vi "VISP Snippet Write.vi"(8 "error in (no error)":errorcluster, 9 "Image Data in":T1, 10 "VI Path (*.vi)":path, 11 "VI Snippet Path (*.png)":path) -> (0 "error out":errorcluster)   [LabVIEW 2019, in "VI Snippet.lvlib"]
doc: "Writes the <b>VI Snippet Path (*.png)</b> image to disk including the embedded <b>VI Path (*.vi)</b> specified (as the \"niVI\" PNG chunk).\n\nCreated by: Ryan Pacini"
uses:
  VI Snippet.lvlib
  <vilib>/picture/picture.llb/imagedata.ctl
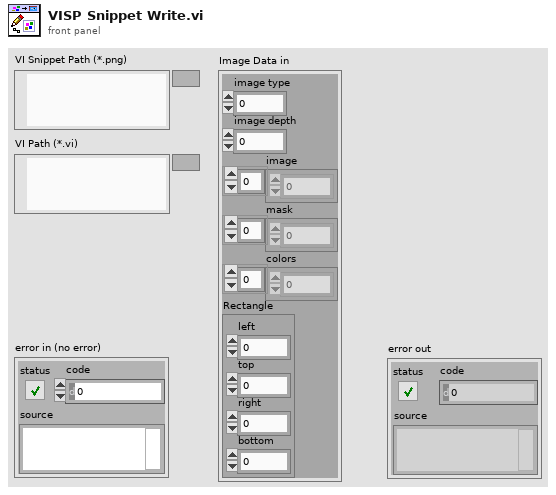
[diagram p1: front panel]
types:
  T1 = typedef "imagedata.ctl" = cluster{"image type":i32, "image depth":i32, "image":u8[], "mask":u8[], "colors":u32[], "Rectangle":cluster{"left":i16, "top":i16, "right":i16, "bottom":i16}}
  T2 = typedef "VI Snippet.lvlib/VISP PNG Chunk.ctl" = cluster{"Length":i32, "Type":string, "Data":string, "CRC":u32}
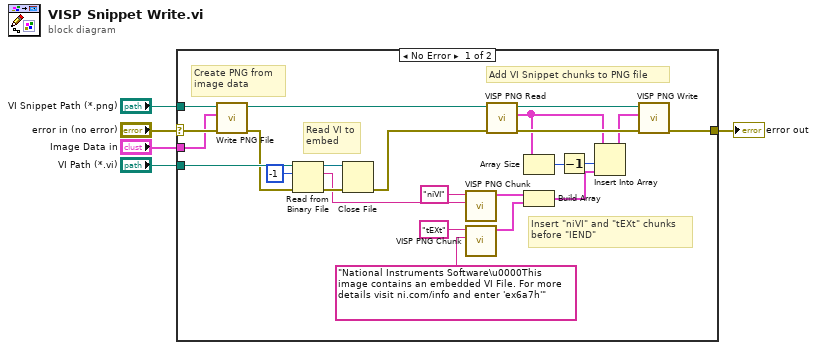
[diagram p0: block diagram]
diagram:
  n1 = case shown="No Error" "error in (no error)" {
    selector: "error in (no error)" -> [w29 w30]
    tunnel: "VI Snippet Path (*.png)" -> [w28 _]
    tunnel: "Image Data in" -> [w27 _]
    tunnel: [w16 w30] -> w3
    tunnel: "VI Path (*.vi)" -> [w15 _]
    frame No Error {
      # "Read VI to\nembed"
      # "Create PNG from\nimage data"
      # "Add VI Snippet chunks to PNG file"
      # "Insert \"niVI\" and \"tEXt\" chunks\nbefore \"IEND\""
      n2 = call <vilib>:"Write PNG File.vi"("error in (no error)"=w29, "image data"=w27, "path to PNG file"=w28) -> ("error out"=w11:errorcluster, "path"=w8:path)  [unwired: 7 in]
      n3 = Read from Binary File(8:w11, 10:-1 ("count (1)"), 11:w15) -> (0:w13:errorcluster, 2:w9:string, 3:w12:refnum<file>)  [unwired: 3 in, 1 out]
      n4 = Close File(refnum=w12, error in=w13) -> (error out=w10:errorcluster)  [unwired: 1 out]
      n5 = call "VISP PNG Chunk.vi"("Data"=w9, "Type"="niVI") -> ("PNG Chunk"=w19:T2)  [unwired: 9 in]
      n6 = call "VISP PNG Chunk.vi"("Data"="National Instruments Software\u0000This image contains an embedded VI File. For more details visit ni.com/info and enter 'ex6a7h'", "Type"="tEXt") -> ("PNG Chunk"=w18:T2)  [unwired: 9 in]
      n7 = call "VISP PNG Read.vi"("error in (no error)"=w10, "Image Path (*.png)"=w8) -> ("error out"=w26:errorcluster, "Chunks"=w7:T2[], "dup Image Path"=w6:path)  [unwired: 7 in]
      n8 = Array Size(array=w7) -> (size(s)=w24:i32)
      n9 = Build Array(w19, w18) -> (w17:T2[])
      n10 = Decrement(x=w24) -> (x-1=w23:i32)
      n11 = Insert Into Array(array=w7, index=w23, new element=w17) -> (w25:T2[])
      n12 = call "VISP PNG Write.vi"("error in (no error)"=w26, "Chunks"=w25, "Image Path (*.png)"=w6) -> ("error out"=w16:errorcluster)  [unwired: 7 in, 1 out]
    }
    frame Error {
    }
  }
  "error out" <- w3
